vi "CodeBlockConcate.vi"(0 "appended path":path, 1 "rm_data_DL":dbl[][](array[numeric]), 2 "Cluster":T1, 3 "rm_len":dbl[](array[numeric]), 4 "error in (no error)":errorcluster caption="错误输入（无错误）") -> (5 "ccbc_data":dbl[](array[numeric]), 6 "error out":errorcluster caption="错误输出")   [LabVIEW 2015]
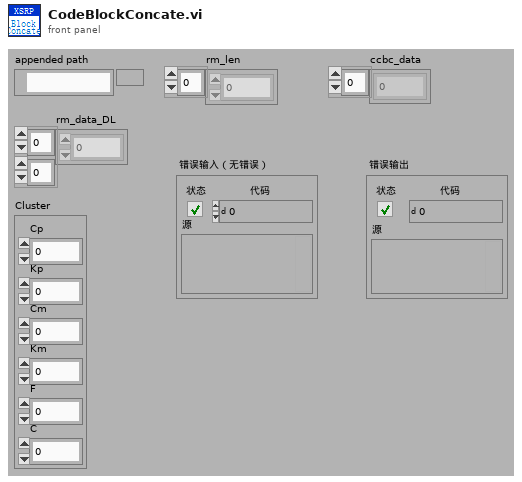
[diagram p1: front panel]
types:
  T1 = cluster{"Cp":dbl, "Kp":dbl, "Cm":dbl, "Km":dbl, "F":dbl, "C":dbl}
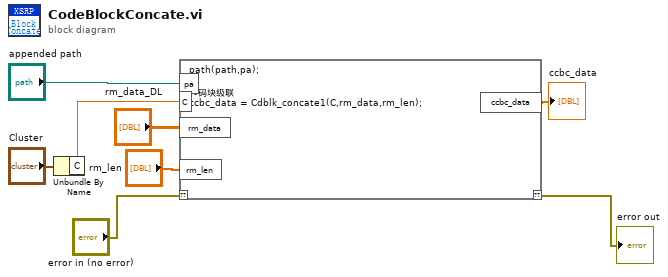
[diagram p0: block diagram]
diagram:
  n1 = Unbundle By Name("Cluster") -> ("C"=w7:dbl)
  n2 = script code="path(path,pa);\n\n%码块级联\nccbc_data = Cdblk_concate1(C,rm_data,rm_len);"("??"="error in (no error)", "pa"="appended path", "rm_data"="rm_data_DL", "rm_len"="rm_len", "C"=w7) -> ("??"=→"error out":errorcluster, "ccbc_data"=→"ccbc_data":dbl[])
